vi "LS234 Send Calibration.vi"() -> ()   [LabVIEW 2021]
uses:
  <vilib>/Analysis/NI_AALPro.lvlib
panel:
  in  "Calibration":string
  in  "Send Calibration":bool
  out "?":cluster{dbl[], dbl[]}[](graph)
  # "(Empty gives dialog)"
  # "Don't Send Calibrations"
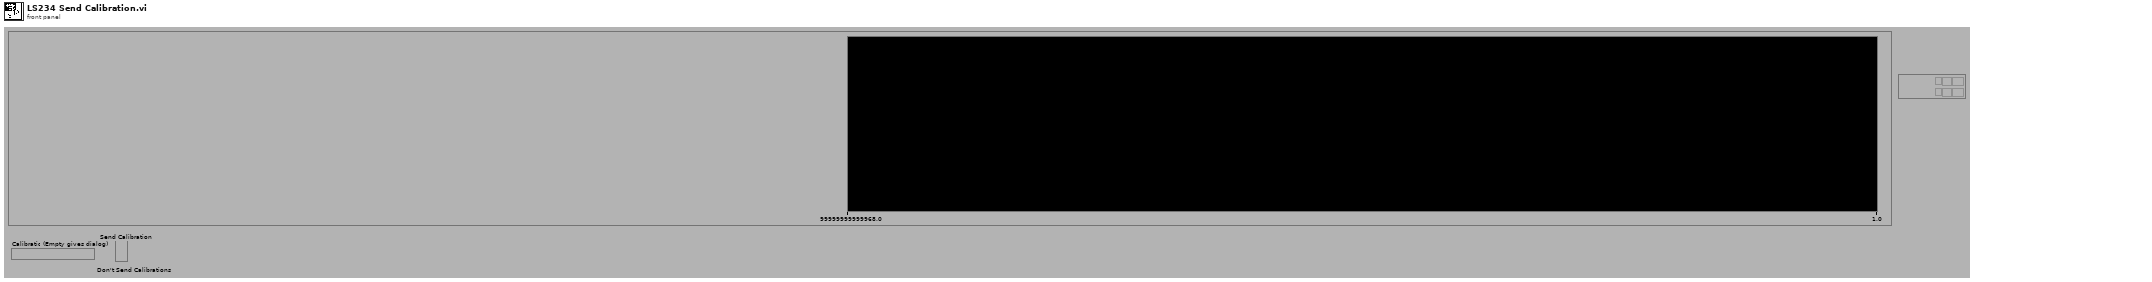
[diagram p1: front panel]
types:
  T1 = cluster{"Temperature":dbl[], "Resistance":dbl[]}[]
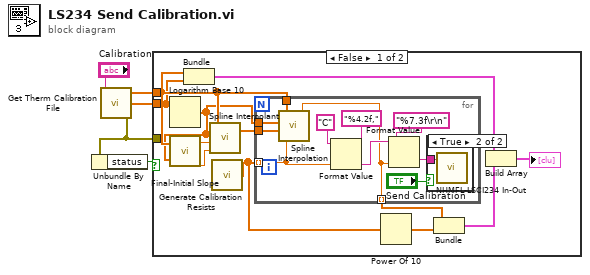
[diagram p0: block diagram]
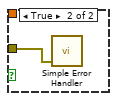
[diagram p3: hidden frame]
diagram:
  n1 = call "Get Therm Calibration File.vi"("Calibration (Empty gives dialog)"="Calibration") -> ("Temperature"=w3:dbl[], "Resistance"=w2:dbl[], "error out"=w4:errorcluster)  [unwired: 1 out]
  n2 = Unbundle By Name(w4) -> ("status"=w5:bool)
  n3 = case shown="False" w5 {
    tunnel: w3 -> [w8 _]
    tunnel: w2 -> [w7 _]
    tunnel: w4 -> [_ w30]
    frame False {
      n4 = Logarithm Base 10(1:w7) -> (0:w6:dbl[])
      n5 = call "Final-Initial Slope.vi"("X Array"=w6, "Y Array"=w8) -> ("Final Slope"=w9:dbl, "Initial Slope"=w10:dbl)
      n6 = Bundle("Temperature"=w8, "Resistance"=w7) -> (w13:cluster{"Temperature":dbl[], "Resistance":dbl[]})  [unwired: 1 in]
      n7 = call <vilib>:"Spline Interpolant.vi"("final boundary"=w9, "initial boundary"=w10, "X"=w6, "Y"=w8) -> ("Interpolant"=w17:dbl[])  [unwired: 1 out]
      n8 = call "Generate Calibration Resists.vi"() -> (0:w16:dbl[])  [unwired: 4 in]
      n9 = for {
        tunnel: w17 -> [w28]
        tunnel: w16 -> [w23] mode=indexing
        tunnel: w6 -> [w27]
        tunnel: w8 -> [w26]
        tunnel: [w20] -> w12 mode=indexing
        n10 = call <vilib>:"Spline Interpolation.vi"("x value"=w23, "Interpolant"=w28, "X"=w27, "Y"=w26) -> ("interpolation value"=w20:dbl)  [unwired: 1 out]
        n11 = Format Value(string ("")="C", format string="%4.2f,", value (0)=w23) -> (output string=w22:string)
        n12 = Format Value(string ("")=w22, format string="%7.3f\r\n", value (0)=w20) -> (output string=w19:string)
        n13 = case shown="True" "Send Calibration" {
          tunnel: w19 -> [_ w29]
          frame False {
          }
          frame True {
            n14 = call "NHMFL-LSCI234 In-Out.vi"("Comand String"=w29) -> ()  [unwired: 1 in, 2 out]
          }
        }
      }
      n15 = Power Of 10(x=w16) -> (10^x=w11:dbl[])
      n16 = Bundle(w12, w11) -> (w15:cluster{dbl[], dbl[]})  [unwired: 1 in]
      n17 = Build Array(w13, w15) -> (→"?":T1)
    }
    frame True {
      n18 = call <vilib>:"Simple Error Handler.vi"("error in (no error)"=w30) -> ()  [unwired: 4 in, 5 out]
    }
  }
